vi "SetMatlabTempParamData.vi"(8 "index in":dbl=-1.0, 10 "Matlab param data":T1[](array[typedef]), 11 "ExperimentID":string) -> (3 "index out":dbl)   [LabVIEW 2017]
uses:
  Types/MatlabDataBundle.ctl
  Types/MatlabDataType.ctl
  <vilib>/Utility/Data Type/Type Definitions/Data Type.ctl
  <vilib>/Utility/Data Type/NI_Data Type.lvlib
panel:
  out "tempMapId":dbl
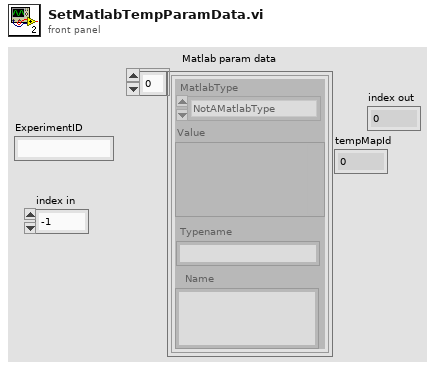
[diagram p1: front panel]
types:
  T1 = typedef "MatlabDataBundle.ctl" = cluster{"MatlabType":T2, "Value":variant, "Name":string, "Typename":string}
  T2 = typedef "MatlabDataType.ctl" = enum16{"NotAMatlabType", "Real", "Complex", "String", "Boolean"}
  T3 = typedef "NI_Data Type.lvlib/Data Type.ctl" = enum8{"Invalid Type", "Void", "I8", "I16", "I32", "I64", "U8", "U16", "U32", "U64", "Single Float", "Double Float", "Extended Float", "Single Complex", "Double Complex", "Extended Complex", "Enum U8", "Enum U16", "Enum U32", "Enum U64", "Single Float With Unit", "Double Float With Unit", "Extended Float With Unit", "Single Complex with Unit", "Double Complex with Unit", "Extended Complex with Unit", "Boolean", "String", "Path", "Picture", "Tag", "Array", "Cluster", "Variant", "LV Variant", "Waveform", "Timestamp", "Digital Waveform", "Digital Data", "ExpressData", "Refnum", "External Data", "VI", "Poly VI", "LabVIEW Class Instance", "Fixed Point"}
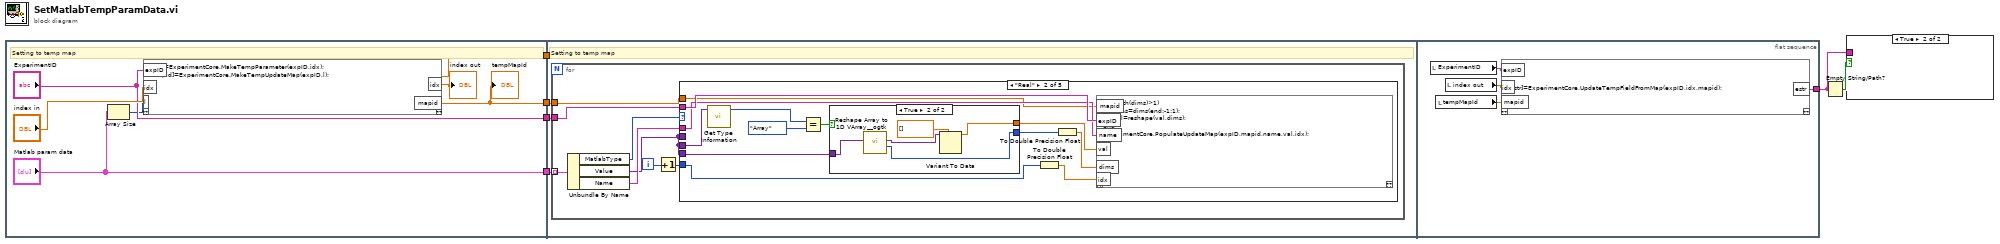
[diagram p0: block diagram]
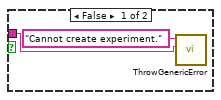
[diagram p2: hidden frame]
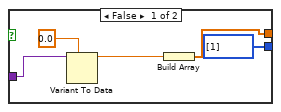
[diagram p4: hidden frame]
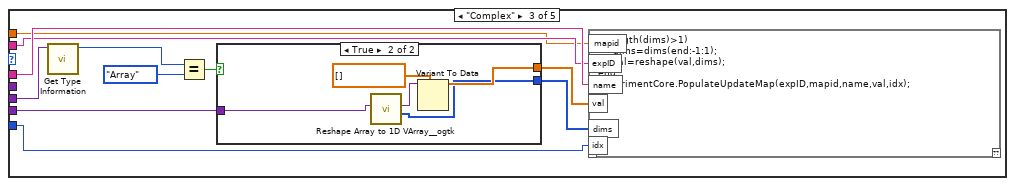
[diagram p5: hidden frame]
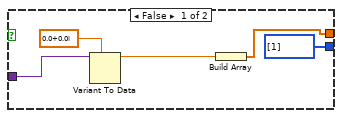
[diagram p6: hidden frame]
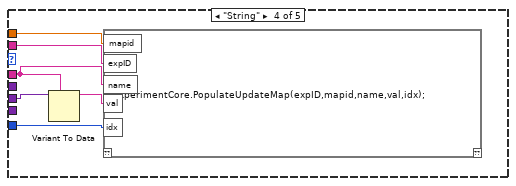
[diagram p7: hidden frame]
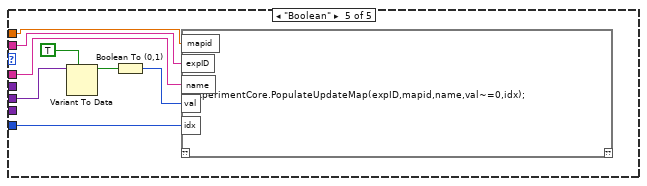
[diagram p8: hidden frame]
diagram:
  n1 = flat-sequence {
    tunnel: [w11] -> w6
    tunnel: ["ExperimentID"] -> w5
    tunnel: ["Matlab param data"] -> w4
    tunnel: [w7] -> w3
    tunnel: w6 -> [_]
    tunnel: w5 -> [w14]
    tunnel: w4 -> [w15]
    tunnel: w3 -> [w13]
    tunnel: [w82] -> w1
    frame #0 {
      # "Setting to temp map"
      n2 = Array Size(array="Matlab param data") -> (size(s)=w8:i32)
      n3 = script code="[idx]=ExperimentCore.MakeTempParameter(expID,idx);\n[mapid]=ExperimentCore.MakeTempUpdateMap(expID,l);"("expID"="ExperimentID", "idx"="index in", "l"=w8) -> ("idx"=w11:dbl, "mapid"=w7:dbl)  [unwired: 1 in, 1 out]
      "index out" <- w11
      "tempMapId" <- w7
    }
    frame #1 {
      # "Setting to temp map"
      n4 = for {
        tunnel: w15 -> [w22] mode=indexing
        tunnel: w14 -> [w23]
        tunnel: w13 -> [w18]
        i -> [w17]
        n5 = Unbundle By Name(w22) -> ("MatlabType"=w21:T2, "Value"=w19:variant, "Name"=w20:string)
        n6 = Increment(x=w17) -> (x+1=w16:i32)
        n7 = case shown="\"Real\"" w21 {
          tunnel: w23 -> [_ w36 w48 w72 w78]
          tunnel: w19 -> [_ w34 w57 w73 w77]
          tunnel: w20 -> [_ w35 w49 w71 w76]
          tunnel: w19 -> [_ _ _ _ _]
          tunnel: w19 -> [_ w29 w53 _ _]
          tunnel: w16 -> [_ w25 w51 w69 w75]
          tunnel: w18 -> [_ w28 w47 w68 w74]
          frame "NotAMatlabType", Default {
          }
          frame "Real" {
            n8 = call <vilib>:"Get Type Information.vi"("Variant"=w34) -> ("Type"=w32:T3)  [unwired: 6 in, 4 out]
            n9 = Equal?(x=w32, y=Data_Type."Array" ("Type")) -> (x = y?=w31:bool)
            n10 = case shown="True" w31 {
              tunnel: [w39 w45] -> w30
              tunnel: w29 -> [w37 w44]
              tunnel: [u32[] [1] ("Size(s)") w43] -> w27
              frame False {
                n11 = Variant To Data(type=0.0, Variant=w37) -> (data=w40:dbl)  [unwired: 1 in, 1 out]
                n12 = Build Array(w40) -> (w39:dbl[])
              }
              frame True {
                n13 = call <userlib>:"Reshape Array to 1D VArray__ogtk.vi"("MultiD Array"=w44) -> ("Size(s)"=w43:u32[], "1D VArray"=w42:variant)  [unwired: 8 in, 1 out]
                n14 = Variant To Data(type=dbl[] [], Variant=w42) -> (data=w45:dbl[])  [unwired: 1 in, 1 out]
              }
            }
            n15 = To Double Precision Float(number=w25) -> (double precision float=w24:dbl)
            n16 = To Double Precision Float(number=w27) -> (double precision float=w26:dbl[])
            n17 = script code="if(length(dims)>1)\n     dims=dims(end:-1:1);\n     val=reshape(val,dims);\nend\nExperimentCore.PopulateUpdateMap(expID,mapid,name,val,idx);"("expID"=w36, "name"=w35, "val"=w30, "mapid"=w28, "dims"=w26, "idx"=w24) -> ()  [unwired: 1 in, 1 out]
          }
          frame "Complex" {
            n18 = call <vilib>:"Get Type Information.vi"("Variant"=w57) -> ("Type"=w55:T3)  [unwired: 6 in, 4 out]
            n19 = Equal?(x=w55, y=Data_Type."Array" ("Type")) -> (x = y?=w54:bool)
            n20 = case shown="True" w54 {
              tunnel: [w61 w66] -> w50
              tunnel: w53 -> [w59 w65]
              tunnel: [u32[] [1] ("Size(s)") w64] -> w52
              frame False {
                n21 = Variant To Data(type=cdb 0.0+0.0i, Variant=w59) -> (data=w62:cdb)  [unwired: 1 in, 1 out]
                n22 = Build Array(w62) -> (w61:cdb[])
              }
              frame True {
                n23 = call <userlib>:"Reshape Array to 1D VArray__ogtk.vi"("MultiD Array"=w65) -> ("Size(s)"=w64:u32[], "1D VArray"=w63:variant)  [unwired: 8 in, 1 out]
                n24 = Variant To Data(type=cdb[] [], Variant=w63) -> (data=w66:cdb[])  [unwired: 1 in, 1 out]
              }
            }
            n25 = script code="if(length(dims)>1)\n     dims=dims(end:-1:1);\n     val=reshape(val,dims);\nend\nExperimentCore.PopulateUpdateMap(expID,mapid,name,val,idx);"("expID"=w48, "name"=w49, "val"=w50, "mapid"=w47, "dims"=w52, "idx"=w51) -> ()  [unwired: 1 in, 1 out]
          }
          frame "String" {
            n26 = Variant To Data(type=w71, Variant=w73) -> (data=w70:string)  [unwired: 1 in, 1 out]
            n27 = script code="ExperimentCore.PopulateUpdateMap(expID,mapid,name,val,idx);"("expID"=w72, "name"=w71, "val"=w70, "mapid"=w68, "idx"=w69) -> ()  [unwired: 1 in, 1 out]
          }
          frame "Boolean" {
            n28 = Variant To Data(type=TRUE, Variant=w77) -> (data=w80:bool)  [unwired: 1 in, 1 out]
            n29 = Boolean To (0,1)(Boolean=w80) -> (0, 1=w79:i16)
            n30 = script code="ExperimentCore.PopulateUpdateMap(expID,mapid,name,val~=0,idx);"("expID"=w78, "name"=w76, "val"=w79, "mapid"=w74, "idx"=w75) -> ()  [unwired: 1 in, 1 out]
          }
        }
      }
    }
    frame #2 {
      n31 = local read "ExperimentID"() -> (w83:string)
      n32 = local read "tempMapId"() -> (w84:dbl)
      n33 = local read "index out"() -> (w85:dbl)
      n34 = script code="[estr]=ExperimentCore.UpdateTempFieldFromMap(expID,idx,mapid);"("expID"=w83, "idx"=w85, "mapid"=w84) -> ("estr"=w82:string)  [unwired: 1 in, 1 out]
    }
  }
  n35 = Empty String/Path?(string/path=w1) -> (empty?=w2:bool)
  n36 = case shown="True" w2 {
    tunnel: w1 -> [w86 _]
    frame False {
      n37 = call "ThrowGenericError.vi"("Error info"=w86, "TheError"="Cannot create experiment.") -> ()  [unwired: 9 in, 1 out]
    }
    frame True {
    }
  }
